vi "collect Device Informations.vi"(4 "error in (no error)":errorcluster caption="Error IN", 5 "close device?":bool=TRUE, 6 "preselection product":enum8{"only Sepia II", "only Solea", "all"}(ring)=enum."all", 7 "PerformRestart":enum8{"no Restart", "Restart"}(ring)) -> (0 "error out":errorcluster caption="Error OUT", 1 "device infos":T1, 2 "Deviceinfo (TXT)":string, 3 "Last Error":T2)   [LabVIEW 2020]
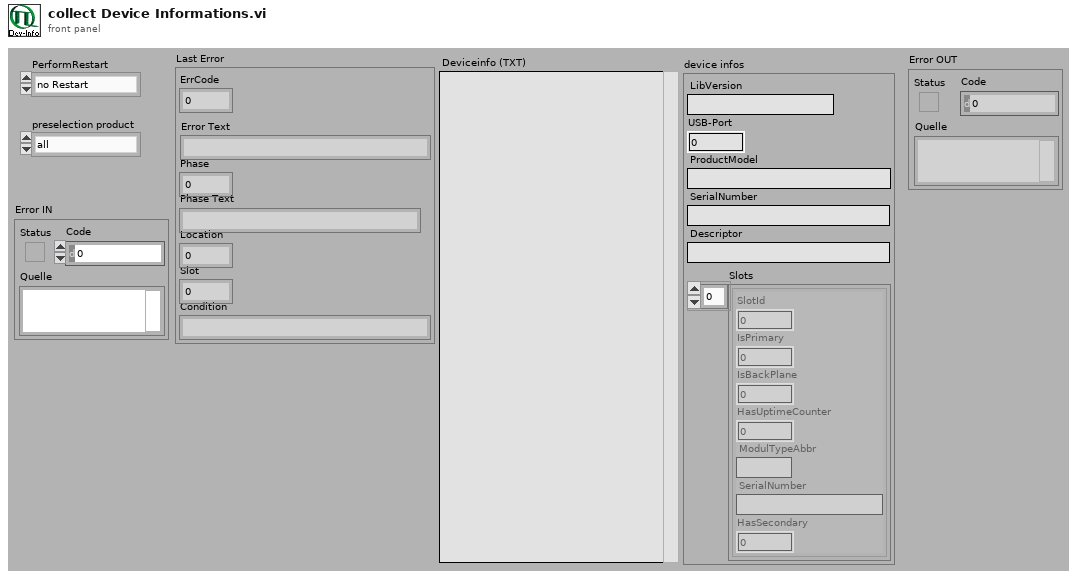
[diagram p1: front panel]
types:
  T1 = cluster{"LibVersion":string, "USB-Port":i32, "ProductModel":string, "SerialNumber":string, "Descriptor":string, "Slots":cluster{"SlotId":i32, "IsPrimary":u8, "IsBackPlane":u8, "HasUptimeCounter":u8, "ModulTypeAbbr":string, "SerialNumber":string, "HasSecondary":i32}[]}
  T2 = cluster{"ErrCode":i32, "Error Text":string, "Phase":i32, "Phase Text":string, "Location":i32, "Slot":i32, "Condition":string}
  T3 = cluster{"SlotId":i32, "IsPrimary":u8, "IsBackPlane":u8, "HasUptimeCounter":u8, "ModulTypeAbbr":string, "SerialNumber":string, "HasSecondary":i32}[]
  T4 = cluster{"DevIdx":i32, "ProductModel":string, "SerialNumber":string}[]
  T5 = cluster{"DevIdx":i32, "ProductModel":string, "SerialNumber":string}
  T6 = cluster{"SlotId":i32, "IsPrimary":u8, "IsBackPlane":u8, "HasUptimeCounter":u8, "ModulTypeAbbr":string, "SerialNumber":string, "HasSecondary":i32}
  T7 = cluster{"SlotId":i32, "IsPrimary":u8, "IsBackPlane":u8, "HasUptimeCounter":u8}
  T8 = cluster{"MainPowerUp":u32, "ActivePowerUp":u32, "ScaledPowerUp":u32}
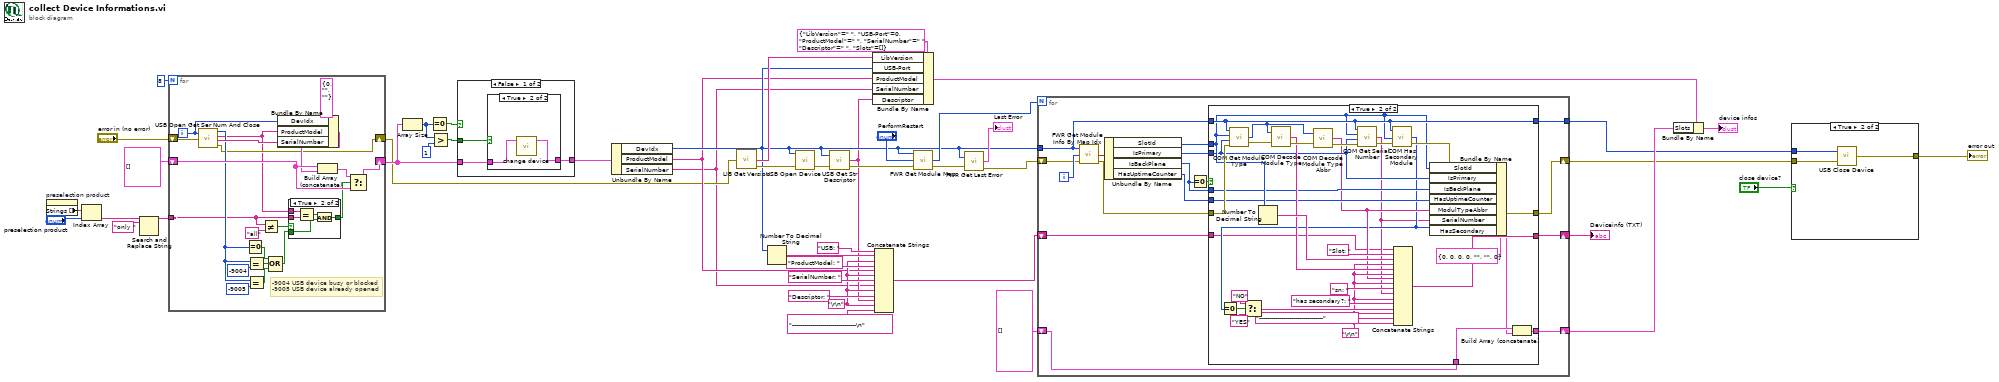
[diagram p0: block diagram]
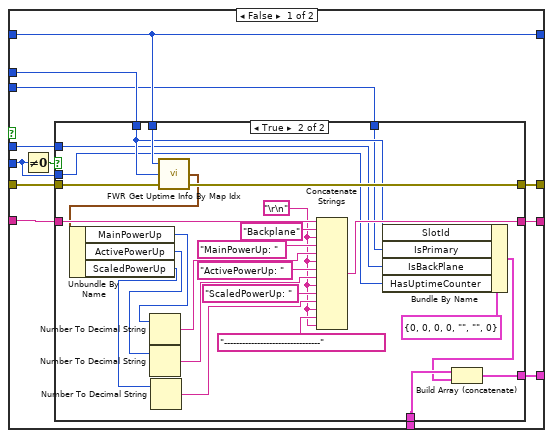
[diagram p3: hidden frame]
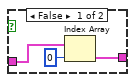
[diagram p5: hidden frame]
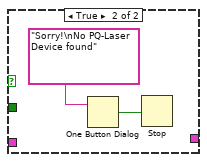
[diagram p6: hidden frame]
diagram:
  w25 = "\r\n"
  n1 = property on="preselection product" class="Enum (strict)"() -> ("Strings []"=w11:string[])  [unwired: 2 in, 2 out]
  n2 = Index Array(array=w11, index="preselection product") -> (element=w9:string)
  n3 = Search and Replace String(input string=w9, search string="only " ("regular expression")) -> (result string=w7:string)  [unwired: 6 in, 3 out]
  n4 = for {
    N: 8 -> [_]
    shift-right: [w63] -> w41
    shift-left: T4 [] -> [w62]
    shift-right: [w53] -> w12
    shift-left: "error in (no error)" -> [w54]
    tunnel: w7 -> [w49]
    i -> [w65]
    # "-9004 USB device busy or blocked\n-9005 USB device already opened"
    n5 = call "USB Open Get Ser Num And Close.vi"("DevIdx"=w65, "error in (no error)"=w54) -> ("function return"=w55:i32, "ProductModel"=w50:string, "SerialNumber"=w66:string, "error out"=w53:errorcluster)
    n6 = Equal To 0?(x=w55) -> (x = 0?=w58:bool)
    n7 = Equal?(x=w55, y=-9004) -> (x = y?=w57:bool)
    n8 = Equal?(x=w55, y=-9005) -> (x = y?=w56:bool)
    n9 = Not Equal?(x=w49, y="all") -> (x != y?=w47:bool)
    n10 = Compound Arithmetic op=OR(w58, w57, w56) -> (w52:bool)
    n11 = Bundle By Name(cluster=T5 {"DevIdx"=0, "ProductModel"="", "SerialNumber"=""} ("input cluster"), "DevIdx"=w65, "ProductModel"=w50, "SerialNumber"=w66) -> (w61:T5)
    n12 = case shown="True" w47 {
      tunnel: w52 -> [w68 w73]
      tunnel: [w68 w72] -> w51
      tunnel: w49 -> [_ w71]
      tunnel: w50 -> [_ w70]
      frame False {
      }
      frame True {
        n13 = Equal?(x=w70, y=w71) -> (x = y?=w69:bool)
        n14 = And(x=w69, y=w73) -> (x .and. y?=w72:bool)
      }
    }
    n15 = Build Array (concatenate)(w62, w61) -> (w64:T4)
    n16 = Select(t=w64, s=w51, f=w62) -> (s? t:f=w63:T4)
  }
  n17 = Array Size(array=w41) -> (size(s)=w1:i32)
  n18 = Equal To 0?(x=w1) -> (x = 0?=w44:bool)
  n19 = Greater?(x=w1, y=1) -> (0:w42:bool)
  n20 = case shown="False" w44 {
    tunnel: w42 -> [w76 _]
    tunnel: w41 -> [w75 _]
    tunnel: [w74 _] -> w40
    frame False {
      n21 = case shown="True" w76 {
        tunnel: w75 -> [w79 w80]
        tunnel: [w77 w81] -> w74
        frame False {
          n22 = Index Array(array=w79, index=0) -> (element=w77:T5)
        }
        frame True {
          n23 = call "change device.vi"("DeviceList"=w80) -> ("device"=w81:T5)  [unwired: 4 in]
        }
      }
    }
    frame True {
      n24 = One Button Dialog(message="Sorry!\nNo PQ-Laser Device found") -> (true=w82:bool)  [unwired: 1 in]
      n25 = Stop(stop? (T)=w82) -> ()
    }
  }
  n26 = Unbundle By Name(w40) -> ("DevIdx"=w20:i32, "ProductModel"=w19:string, "SerialNumber"=w2:string)
  n27 = call "LIB Get Version.vi"("error in (no error)"=w12) -> ("LibVersion"=w21:string, "error out"=w31:errorcluster)  [unwired: 1 out]
  n28 = Number To Decimal String(number=w20) -> (decimal integer string=w29:string)  [unwired: 1 in]
  n29 = call "USB Open Device.vi"("error in (no error)"=w31, "DevIdx"=w20) -> ("error out"=w39:errorcluster)  [unwired: 2 in, 3 out]
  n30 = call "USB Get Str Descriptor.vi"("DevIdx"=w20, "error in (no error)"=w39) -> ("Descriptor"=w18:string, "error out"=w37:errorcluster)  [unwired: 1 out]
  n31 = Bundle By Name(cluster=T1 {"LibVersion"=" ", "USB-Port"=0, "ProductModel"=" ", "SerialNumber"=" ", "Descriptor"=" ", "Slots"=[]}, "LibVersion"=w21, "USB-Port"=w20, "ProductModel"=w19, "SerialNumber"=w2, "Descriptor"=w18) -> (w17:T1)
  n32 = Concatenate Strings("USB: ", w29, w25, "ProductModel: ", w19, w25, "SerialNumber: ", w2, w25, "Descriptor: ", w18, w25, "--------------------------------\n") -> (w23:string)
  n33 = call "FWR Get Module Map.vi"("error in (no error)"=w37, "PerformRestart"="PerformRestart", "DevIdx"=w20) -> ("error out"=w36:errorcluster, "ModuleCount"=w34:i32)  [unwired: 1 out]
  n34 = call "FWR Get Last Error.vi"("DevIdx"=w20, "error in (no error)"=w36) -> ("Last Error"=→"Last Error":T2, "error out"=w33:errorcluster)  [unwired: 1 out]
  n35 = for {
    N: w34 -> [_]
    tunnel: w20 -> [w96]
    shift-right: [w84] -> w6
    shift-left: w33 -> [w98]
    shift-right: [w92] -> w32
    shift-left: w23 -> [w93]
    tunnel: [w91] -> w4
    shift-right: [w86] -> w14
    shift-left: T3 [] -> [w85]
    i -> [w99]
    n36 = call "FWR Get Module Info By Map Idx.vi"("error in (no error)"=w98, "MapIdx"=w99, "DevIdx"=w96) -> ("error out"=w97:errorcluster, "FWR Module Info"=w89:T7)  [unwired: 1 out]
    n37 = Unbundle By Name(w89) -> ("SlotId"=w95:i32, "IsPrimary"=w94:u8, "IsBackPlane"=w88:u8, "HasUptimeCounter"=w87:u8)
    n38 = Equal To 0?(x=w88) -> (x = 0?=w90:bool)
    n39 = case shown="True" w90 {
      tunnel: w97 -> [w109 w171]
      tunnel: w96 -> [w110 w156]
      tunnel: w95 -> [w111 w152]
      tunnel: w94 -> [w104 w151]
      tunnel: [w108 w153] -> w84
      tunnel: w93 -> [w107 w141]
      tunnel: [w106 w164] -> w92
      tunnel: [w110 w156] -> w91
      tunnel: w88 -> [w103 w150]
      tunnel: w87 -> [w100 w149]
      tunnel: [w102 w144] -> w86
      tunnel: w85 -> [w101 w145]
      frame False {
        n40 = Not Equal To 0?(x=w100) -> (x != 0?=w105:bool)
        n41 = case shown="True" w105 {
          tunnel: w111 -> [_ w121]
          tunnel: w110 -> [_ w140]
          tunnel: w109 -> [w114 w139]
          tunnel: [w114 w138] -> w108
          tunnel: w107 -> [w113 w137]
          tunnel: [w113 w136] -> w106
          tunnel: w104 -> [_ w120]
          tunnel: w103 -> [_ w116]
          tunnel: w100 -> [_ w119]
          tunnel: [w112 w118] -> w102
          tunnel: w101 -> [w112 w117]
          frame False {
          }
          frame True {
            w125 = "\r\n"
            n42 = call "FWR Get Uptime Info By Map Idx.vi"("error in (no error)"=w139, "MapIdx"=w121, "DevIdx"=w140) -> ("error out"=w138:errorcluster, "FWR Uptime Info"=w134:T8)  [unwired: 1 out]
            n43 = Unbundle By Name(w134) -> ("MainPowerUp"=w132:u32, "ActivePowerUp"=w124:u32, "ScaledPowerUp"=w123:u32)
            n44 = Number To Decimal String(number=w132) -> (decimal integer string=w131:string)  [unwired: 1 in]
            n45 = Number To Decimal String(number=w124) -> (decimal integer string=w129:string)  [unwired: 1 in]
            n46 = Number To Decimal String(number=w123) -> (decimal integer string=w127:string)  [unwired: 1 in]
            n47 = Concatenate Strings(w137, "Backplane" ("string"), w125, "MainPowerUp: " ("string"), w131, w125, "ActivePowerUp: " ("string"), w129, w125, "ScaledPowerUp: " ("string"), w127, w125, "--------------------------------" ("string"), w125) -> (w136:string)
            n48 = Bundle By Name(cluster=T6 {"SlotId"=0, "IsPrimary"=0, "IsBackPlane"=0, "HasUptimeCounter"=0, "ModulTypeAbbr"="", "SerialNumber"="", "HasSecondary"=0}, "SlotId"=w121, "IsPrimary"=w120, "IsBackPlane"=w116, "HasUptimeCounter"=w119) -> (w115:T6)
            n49 = Build Array (concatenate)(w117, w115) -> (w118:T3)
          }
        }
      }
      frame True {
        w154 = "\r\n"
        n50 = call "COM Get Module Type.vi"("error in (no error)"=w171, "GetPrimary"=w151, "SlotId"=w152, "DevIdx"=w156) -> ("error out"=w172:errorcluster, "ModuleType"=w163:i32)  [unwired: 1 out]
        n51 = Number To Decimal String(number=w152) -> (decimal integer string=w167:string)  [unwired: 1 in]
        n52 = call "COM Decode Module Type.vi"("ModuleType"=w163, "error in (no error)"=w172) -> ("ModulType"=w166:string, "error out"=w170:errorcluster)  [unwired: 1 out]
        n53 = call "COM Decode Module Type Abbr.vi"("ModuleType"=w163, "error in (no error)"=w170) -> ("ModulTypeAbbr"=w148:string, "error out"=w169:errorcluster)  [unwired: 1 out]
        n54 = call "COM Get Serial Number.vi"("error in (no error)"=w169, "GetPrimary"=w151, "SlotId"=w152, "DevIdx"=w156) -> ("error out"=w162:errorcluster, "SerialNumber"=w142:string)  [unwired: 1 out]
        n55 = call "COM Has Secondary Module.vi"("error in (no error)"=w162, "SlotId"=w152, "DevIdx"=w156) -> ("error out"=w153:errorcluster, "HasSecondary"=w147:i32)  [unwired: 1 out]
        n56 = Equal To 0?(x=w147) -> (x = 0?=w160:bool)
        n57 = Select(t="NO" ("string"), s=w160, f="YES" ("string")) -> (s? t:f=w159:string)
        n58 = Concatenate Strings(w141, "Slot: ", w167, w154, w166, w154, w148, w154, "sn: " ("string"), w142, w154, "has secondary?: " ("string"), w159, w154, "--------------------------------" ("string"), w154) -> (w164:string)
        n59 = Bundle By Name(cluster=T6 {"SlotId"=0, "IsPrimary"=0, "IsBackPlane"=0, "HasUptimeCounter"=0, "ModulTypeAbbr"="", "SerialNumber"="", "HasSecondary"=0}, "SlotId"=w152, "IsPrimary"=w151, "IsBackPlane"=w150, "HasUptimeCounter"=w149, "ModulTypeAbbr"=w148, "SerialNumber"=w142, "HasSecondary"=w147) -> (w143:T6)
        n60 = Build Array (concatenate)(w145, w143) -> (w144:T3)
      }
    }
  }
  "Deviceinfo (TXT)" <- w32
  n61 = Bundle By Name(cluster=w17, "Slots"=w14) -> (→"device infos":T1)
  n62 = case shown="True" "close device?" {
    tunnel: w6 -> [w173 w176]
    tunnel: [w173 w175] -> w5
    tunnel: w4 -> [_ w174]
    frame False {
    }
    frame True {
      n63 = call "USB Close Device.vi"("error in (no error)"=w176, "DevIdx"=w174) -> ("error out"=w175:errorcluster)
    }
  }
  "error out" <- w5
